vi "Initialize ROV Test.vi"(8 "error in (no error)":errorcluster) -> (0 "error out":errorcluster, 3 "ROV Host.lvclass":refnum<class "ROV Host.lvclass">)   [LabVIEW 2012, in "ROV Host.lvclass"]
uses:
  ROV Host.lvclass
  ROV Host.lvclass/ROV Host.ctl
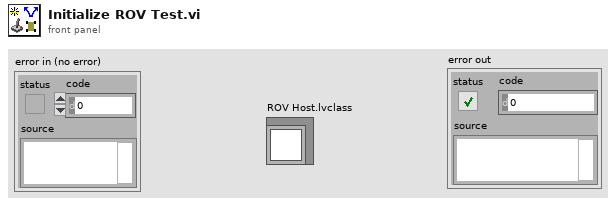
[diagram p1: front panel]
types:
  T1 = typedef "NI_Robotics_Steering Class Types.lvlib/Mecanum Steering Frame.ctl" = refnum<class "NI_Robotics_Mecanum Steering Frame.lvclass">
  T2 = typedef "NI_Robotics_Steering Class Types.lvlib/Differential Steering Frame.ctl" = refnum<class "NI_Robotics_Differential Steering Frame.lvclass">
  T3 = cluster{"mecanum steering frame out":T1, "differential steering frame out":T2}
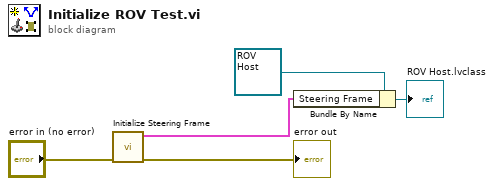
[diagram p0: block diagram]
diagram:
  n1 = call "Initialize Steering Frame.vi"("error in (no error)"="error in (no error)") -> ("error out"=→"error out":errorcluster, "Steering Frame out"=w4:T3)  [unwired: 9 in]
  n2 = Bundle By Name(cluster=refnum<class "ROV Host.lvclass"> refnum ("ROV Host.lvclass"), "Steering Frame"=w4) -> (→"ROV Host.lvclass":refnum<class "ROV Host.lvclass">)
